vi "Introspection Core.vi"(8 "error in (no error)":errorcluster, 11 "CS++MCS in":refnum<class "CS++MCS.lvclass">) -> (0 "error out":errorcluster, 2 "CS++Messages":refnum<class "Message.lvclass">[](array[class]), 3 "CS++MCS out":refnum<class "CS++MCS.lvclass">)   [LabVIEW 2016, in "CS++MCS.lvlib" / "CS++MCS.lvclass"]
doc: "This vi delivers a list with all messages this actor reacts to. \n\nNote that all inherited classes have to overwrite it."
uses:
  CS++MCS.lvclass
  <vilib>/ActorFramework/Message/Message.lvclass
  CS++MCS Messages/Clear Records Msg/Clear Records Msg.lvclass
  C:/Program Files (x86)/National Instruments/LabVIEW 2016/vi.lib/ActorFramework/Message/Message.lvclass
  CS++MCS Messages/Read Data Msg/Read Data Msg.lvclass
  CS++MCS Messages/Start Scan Msg/Start Scan Msg.lvclass
  CS++MCS Messages/Stop Scan Msg/Stop Scan Msg.lvclass
  CS++MCS Messages/Configure BinWidth Msg/Configure BinWidth Msg.lvclass
  CS++MCS Messages/Configure DisLevel Msg/Configure DisLevel Msg.lvclass
  CS++MCS Messages/Configure DisSlope Msg/Configure DisSlope Msg.lvclass
  CS++MCS Messages/Configure NofBins Msg/Configure NofBins Msg.lvclass
  CS++MCS Messages/Configure NofRecords Msg/Configure NofRecords Msg.lvclass
  CS++MCS Messages/Configure TrigLevel Msg/Configure TrigLevel Msg.lvclass
  CS++MCS Messages/Configure TrigSlope Msg/Configure TrigSlope Msg.lvclass
  CSPP_Core/Actors/CS++DeviceActor/CS++DeviceActor.lvclass
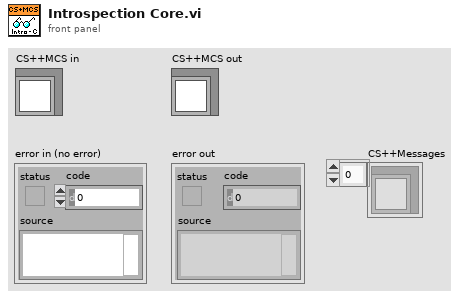
[diagram p1: front panel]
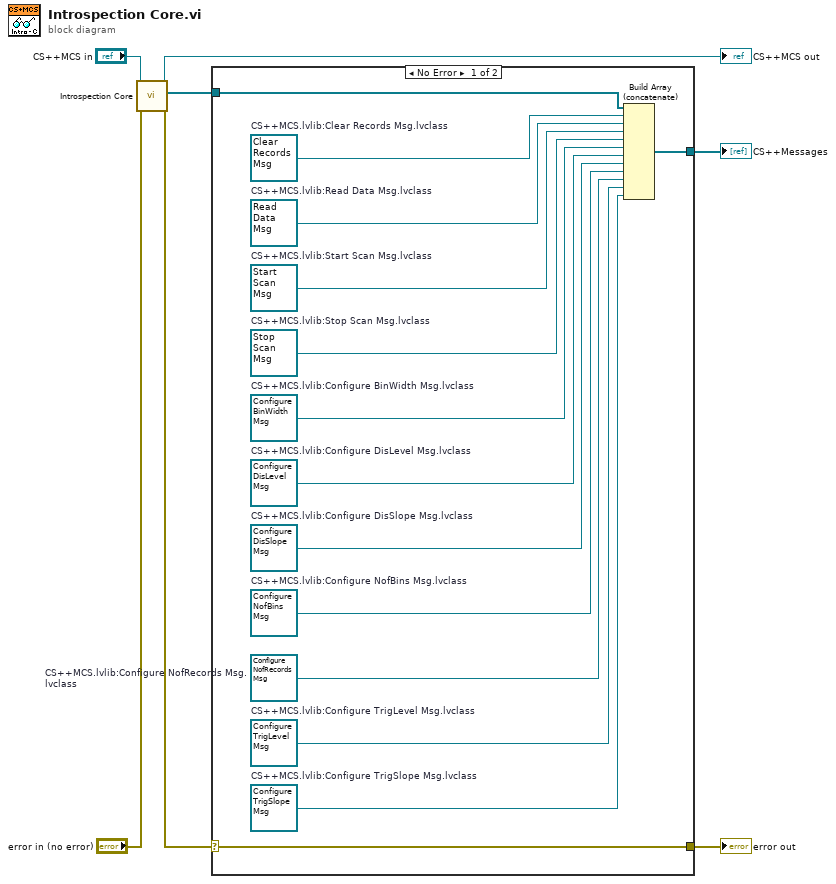
[diagram p0: block diagram]
diagram:
  n1 = call-parent "Introspection Core.vi"("error in (no error)"="error in (no error)", "CS++DeviceActor in"="CS++MCS in") -> ("error out"=w4:errorcluster, "CS++Messages"=w2:refnum<class "Message.lvclass">[], "CS++DeviceActor out"=→"CS++MCS out":refnum<class "CS++MCS.lvclass">)  [unwired: 7 in]
  n2 = case shown="No Error" w4 {
    selector: w4 -> [w21 w23]
    tunnel: [w21 w23] -> w3
    tunnel: w2 -> [w20 w22]
    tunnel: [w19 w22] -> w1
    frame No Error {
      w8 = refnum<class "Configure TrigSlope Msg.lvclass"> refnum  # CS++MCS.lvlib:Configure TrigSlope Msg.lvclass
      w9 = refnum<class "Configure TrigLevel Msg.lvclass"> refnum  # CS++MCS.lvlib:Configure TrigLevel Msg.lvclass
      w10 = refnum<class "Configure NofRecords Msg.lvclass"> refnum  # CS++MCS.lvlib:Configure NofRecords Msg.lvclass
      w11 = refnum<class "Configure NofBins Msg.lvclass"> refnum  # CS++MCS.lvlib:Configure NofBins Msg.lvclass
      w12 = refnum<class "Configure DisSlope Msg.lvclass"> refnum  # CS++MCS.lvlib:Configure DisSlope Msg.lvclass
      w13 = refnum<class "Configure DisLevel Msg.lvclass"> refnum  # CS++MCS.lvlib:Configure DisLevel Msg.lvclass
      w14 = refnum<class "Configure BinWidth Msg.lvclass"> refnum  # CS++MCS.lvlib:Configure BinWidth Msg.lvclass
      w15 = refnum<class "Stop Scan Msg.lvclass"> refnum  # CS++MCS.lvlib:Stop Scan Msg.lvclass
      w16 = refnum<class "Start Scan Msg.lvclass"> refnum  # CS++MCS.lvlib:Start Scan Msg.lvclass
      w17 = refnum<class "Read Data Msg.lvclass"> refnum  # CS++MCS.lvlib:Read Data Msg.lvclass
      w18 = refnum<class "Clear Records Msg.lvclass"> refnum  # CS++MCS.lvlib:Clear Records Msg.lvclass
      n3 = Build Array (concatenate)(w20, w18, w17, w16, w15, w14, w13, w12, w11, w10, w9, w8) -> (w19:refnum<class "Message.lvclass">[])
    }
    frame Error {
    }
  }
  "error out" <- w3
  "CS++Messages" <- w1
